vi "ErrorDataReceivedEvent_CallbackVI.vi"(4 "User Parameter":variant, 5 "Event Data":cluster{"sender":refnum<k24>, "e":refnum<k24>}, 6 "Control Ref":refnum<k24>, 7 "Event Common Data":T1) -> ()   [LabVIEW 2017]
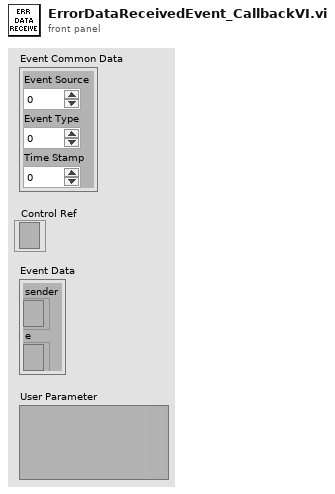
[diagram p1: front panel]
types:
  T1 = cluster{"Event Source":i32, "Event Type":u32, "Time Stamp":u32}
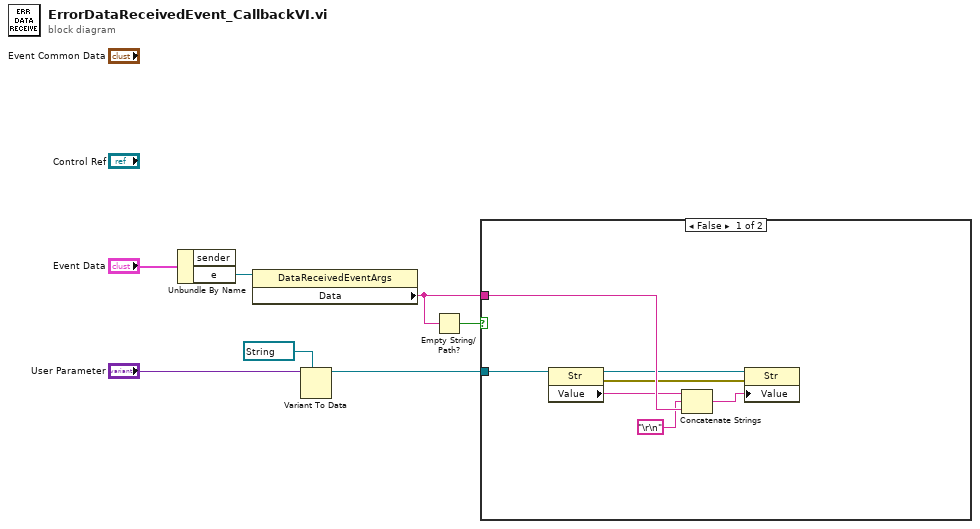
[diagram p0: block diagram]
diagram:
  n1 = Unbundle By Name("Event Data") -> ("e"=w6:refnum<k24>)  [unwired: 1 out]
  n2 = property class="DataReceivedEventArgs"(reference=w6) -> ("Data"=w4:string)  [unwired: 1 in, 2 out]
  n3 = Variant To Data(type=refnum<vi> refnum ("String Ref"), Variant="User Parameter") -> (data=w1:refnum<vi>)  [unwired: 1 in, 1 out]
  n4 = Empty String/Path?(string/path=w4) -> (empty?=w5:bool)
  n5 = case shown="False" w5 {
    tunnel: w4 -> [w13 _]
    tunnel: w1 -> [w14 _]
    frame False {
      n6 = property class="Str"(reference=w14) -> (reference out=w11:refnum<vi>, error out=w10:errorcluster, "Value"=w12:string)  [unwired: 1 in]
      n7 = Concatenate Strings(w12, "\r\n", w13) -> (w9:string)
      n8 = property class="Str"(reference=w11, error in=w10, "Value"=w9) -> ()  [unwired: 2 out]
    }
    frame True {
    }
  }
